vi "Remove State (from Dictionaries).vi"(8 "error in":errorcluster, 10 "state":string, 11 "routing channel in":T1 format="%.0x") -> (0 "error out":errorcluster, 3 "routing channel out":T1=18446744073709551615 format="%.0x")   [LabVIEW 2020, in "Routing and Faulting Scripting.lvlib"]
uses:
  Routing and Faulting Scripting.lvlib
  <vilib>/NI VeriStand/Custom Device API/Custom Device Item Ref.ctl
  NationalInstruments.VeriStand.SystemDefinitionAPI
  Constants/Scripting Constants.vi
  <vilib>/Utility/error.llb/Error Cluster From Error Code.vi
  <vilib>/NI VeriStand/Custom Device API/Custom Device API.lvlib
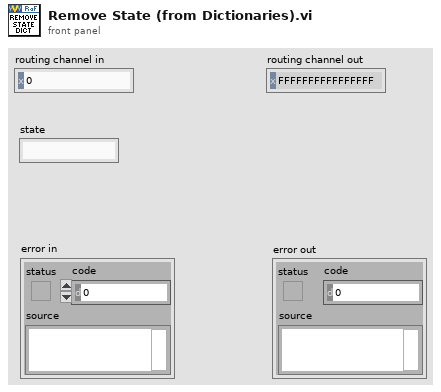
[diagram p1: front panel]
types:
  T1 = typedef "Custom Device API.lvlib/Custom Device Item Ref.ctl" = u64
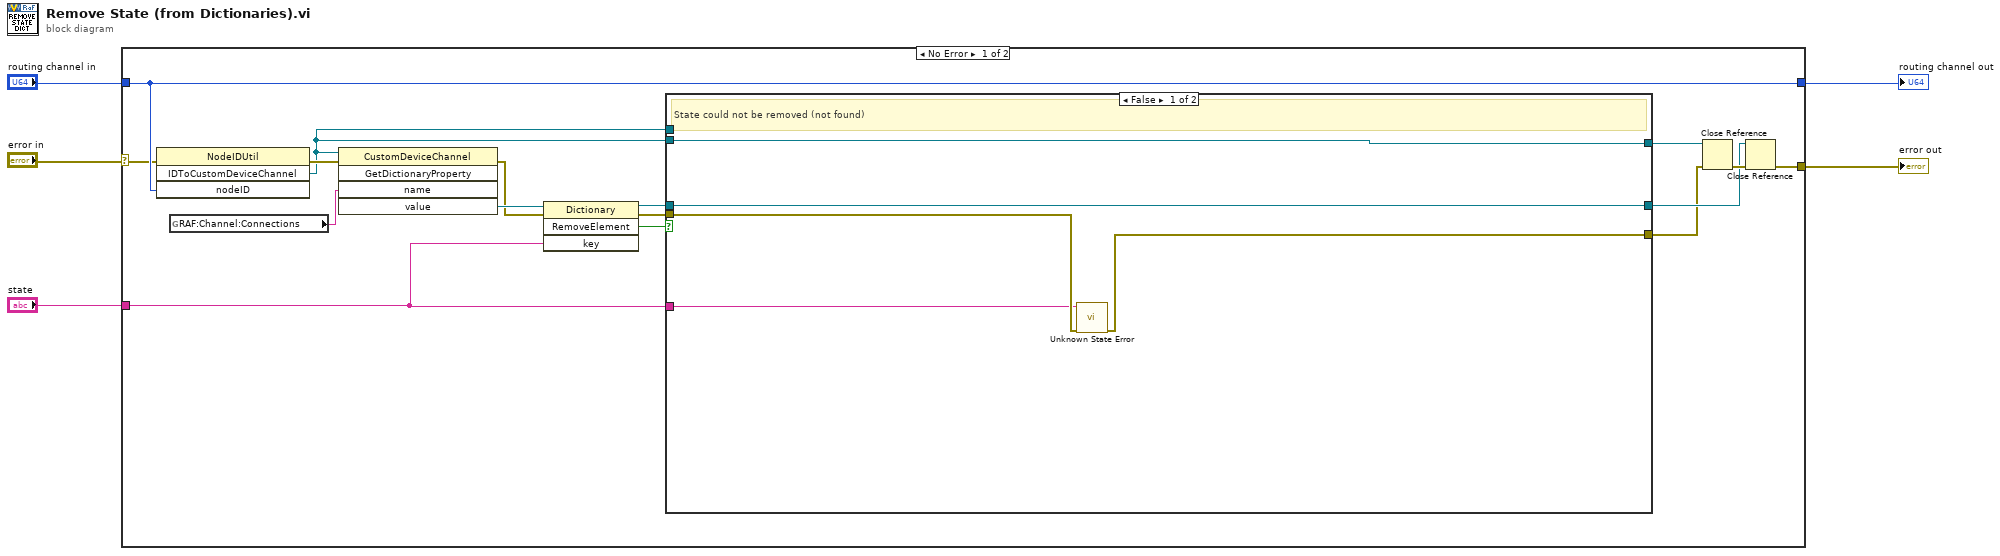
[diagram p0: block diagram]
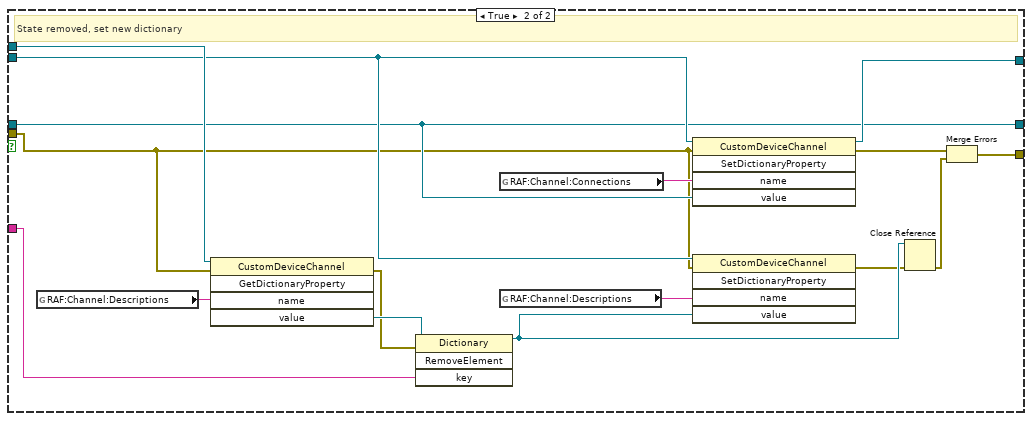
[diagram p2: hidden frame]
diagram:
  n1 = case shown="No Error" "error in" {
    selector: "error in" -> [w18 w44]
    tunnel: [w6 w44] -> w4
    tunnel: "routing channel in" -> [w19 w43]
    tunnel: [w19 w43] -> w2
    tunnel: "state" -> [w8 _]
    frame No Error {
      n2 = invoke class="NodeIDUtil" method="IDToCustomDeviceChannel"(error in=w18, "nodeID"=w19) -> (error out=w20:errorcluster, "IDToCustomDeviceChannel"=w7:refnum<k24>)  [unwired: 2 in, 2 out]
      n3 = global read "Scripting Constants.vi" "RAF:Channel:Connections"() -> (w9:string)
      n4 = invoke class="CustomDeviceChannel" method="GetDictionaryProperty"(reference=w7, error in=w20, "name"=w9) -> (error out=w16:errorcluster, "value"=w17:refnum<k24>)  [unwired: 2 in, 3 out]
      n5 = invoke class="Dictionary" method="RemoveElement"(reference=w17, error in=w16, "key"=w8) -> (reference out=w13:refnum<k24>, error out=w14:errorcluster, "RemoveElement"=w15:bool)  [unwired: 1 in, 1 out]
      n6 = case shown="False" w15 {
        tunnel: w14 -> [w24 w30]
        tunnel: [w23 w32] -> w11
        tunnel: w13 -> [w26 w31]
        tunnel: [w26 w31] -> w12
        tunnel: w7 -> [w25 w34]
        tunnel: [w25 w42] -> w10
        tunnel: w8 -> [w22 w36]
        tunnel: w7 -> [_ w37]
        frame False {
          # "State could not be removed (not found)"
          n7 = call "Unknown State Error.vi"("error in (no error)"=w24, "state"=w22) -> ("error out"=w23:errorcluster)  [unwired: 9 in]
        }
        frame True {
          # "State removed, set new dictionary"
          n8 = global read "Scripting Constants.vi" "RAF:Channel:Descriptions"() -> (w40:string)
          n9 = invoke class="CustomDeviceChannel" method="GetDictionaryProperty"(reference=w37, error in=w30, "name"=w40) -> (error out=w38:errorcluster, "value"=w39:refnum<k24>)  [unwired: 2 in, 3 out]
          n10 = invoke class="Dictionary" method="RemoveElement"(reference=w39, error in=w38, "key"=w36) -> (reference out=w29:refnum<k24>)  [unwired: 1 in, 3 out]
          n11 = global read "Scripting Constants.vi" "RAF:Channel:Connections"() -> (w41:string)
          n12 = global read "Scripting Constants.vi" "RAF:Channel:Descriptions"() -> (w35:string)
          n13 = invoke class="CustomDeviceChannel" method="SetDictionaryProperty"(reference=w34, error in=w30, "name"=w41, "value"=w31) -> (reference out=w42:refnum<k24>, error out=w33:errorcluster)  [unwired: 1 in, 3 out]
          n14 = invoke class="CustomDeviceChannel" method="SetDictionaryProperty"(reference=w34, error in=w30, "name"=w35, "value"=w29) -> (error out=w28:errorcluster)  [unwired: 1 in, 4 out]
          n15 = Close Reference(reference=w29, error in (no error)=w28) -> (error out=w27:errorcluster)
          n16 = Merge Errors(w33, w27) -> (w32:errorcluster)
        }
      }
      n17 = Close Reference(reference=w10, error in (no error)=w11) -> (error out=w21:errorcluster)
      n18 = Close Reference(reference=w12, error in (no error)=w21) -> (error out=w6:errorcluster)
    }
    frame Error {
    }
  }
  "routing channel out" <- w2
  "error out" <- w4
